vi "FTW-Actor-Tag-Set.vi"(0 "FTW-ActorInstance In":refnum<class "FTW-ActorInstance.lvclass">, 7 "Tag Object":variant, 11 "error in":errorcluster) -> (4 "FTW-ActorInstance Out":refnum<class "FTW-ActorInstance.lvclass">, 15 "error out":errorcluster)   [LabVIEW 2015, in "FTW-ActorInstance.lvclass"]
uses:
  FTW-ActorInstance.lvclass
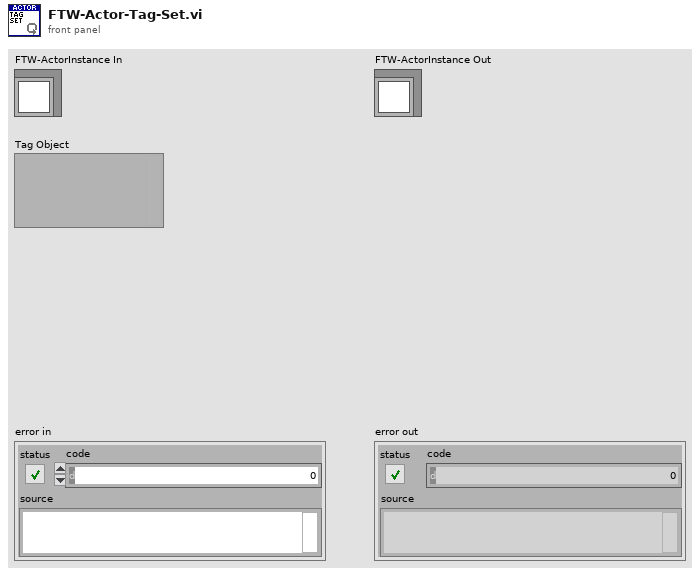
[diagram p1: front panel]
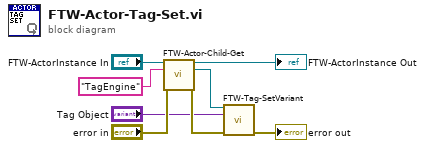
[diagram p0: block diagram]
diagram:
  n1 = call "FTW-Actor-Child-Get.vi"("FTW-ActorInstance In"="FTW-ActorInstance In", "Connector Name"="TagEngine", "error in"="error in") -> ("FTW-ActorInstance Out"=→"FTW-ActorInstance Out":refnum<class "FTW-ActorInstance.lvclass">, "FTW Actor Connector"=w6:refnum<class "FTW-ActorConnector.lvclass">, "error out"=w7:errorcluster)  [unwired: 10 in]
  n2 = call "FTW-Tag-SetVariant.vi"("FTW Actor Connector In"=w6, "Tag Object"="Tag Object", "error in (no error)"=w7) -> ("error out"=→"error out":errorcluster)  [unwired: 10 in, 2 out]
